vi "libdaq_device_get_name.vi"(0 "error in (no error)":errorcluster, 4 "device_index":u32) -> (14 "error out":errorcluster, 18 "device_name":string)   [LabVIEW 2010, in "libdaqVI.lvlib"]
doc: "通过设备索引号获取设备的名称"
uses:
  libdaqVI.lvlib
  dll/daqlib.dll
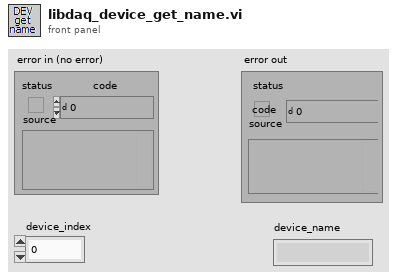
[diagram p1: front panel]
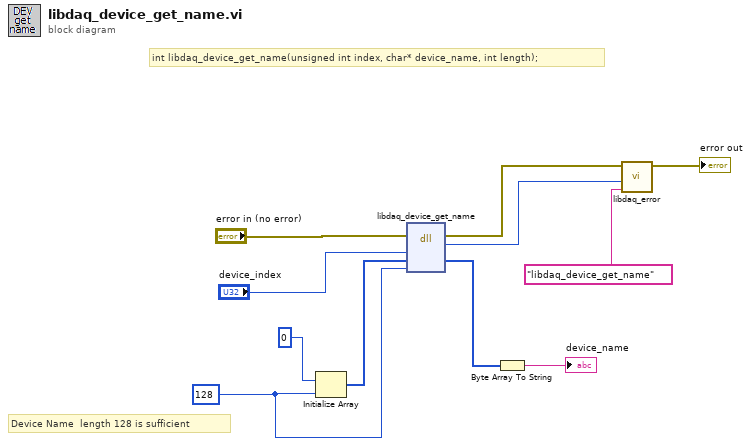
[diagram p0: block diagram]
diagram:
  w8 = 128 ("name_length")
  # "Device Name  length 128 is sufficient"
  # "int libdaq_device_get_name(unsigned int index, char* device_name, int length);"
  n1 = Initialize Array(i8 0, w8) -> (w7:i8[])
  n2 = dll-call lib="E:/Product/Example/DAQ-USB3212/Labview/labview_2010/libdaqVI/dll/daqlib.dll" fn="libdaq_device_get_name"(error in="error in (no error)", "device_index"="device_index", "device_name"=w7, "length"=w8) -> (error out=w4:errorcluster, "return type"=w1:i32, "device_name"=w6:u8[])  [unwired: 4 in, 1 out]
  n3 = Byte Array To String(unsigned byte array=w6) -> (string=→"device_name":string)
  n4 = call "libdaq_error.vi"("error source"="libdaq_device_get_name", "error code"=w1, "错误输入（无错误）"=w4) -> ("错误输出"=→"error out":errorcluster)  [unwired: 8 in]
